vi "Initialize.vi"(8 "error in (no error)":errorcluster caption="错误输入（无错误）", 10 "VISA资源名称":refnum<visa-resource-name>, 11 "34461A 输入":refnum<class "34461A.lvclass">) -> (0 "error out":errorcluster caption="错误输出", 3 "34461A 输出":refnum<class "34461A.lvclass">)   [LabVIEW 2020, in "34461A.lvlib" / "34461A.lvclass"]
uses:
  34461A.lvclass
  <instrlib>/Agilent 3446X Series/Agilent 3446X Series.lvlib
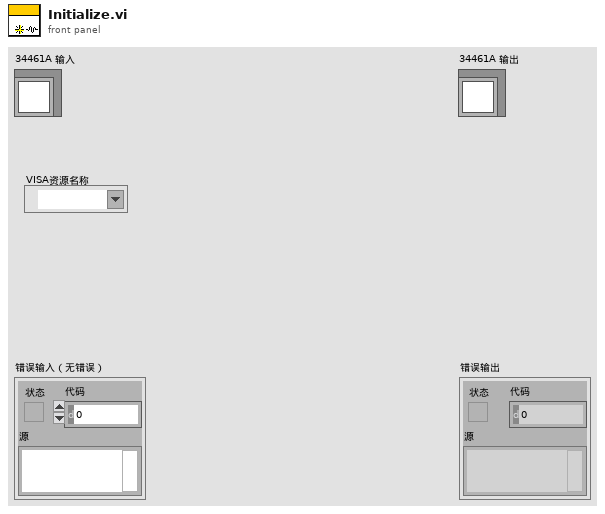
[diagram p1: front panel]
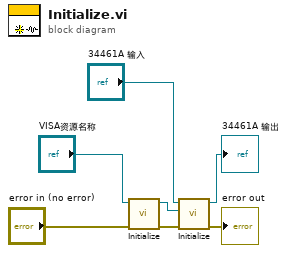
[diagram p0: block diagram]
diagram:
  n1 = call <instrlib>:"Initialize.vi"("error in (no error)"="error in (no error)", "VISA resource name"="VISA资源名称") -> ("error out"=w2:errorcluster, "VISA resource name out"=w1:refnum<visa-resource-name>)  [unwired: 8 in]
  n2 = call-parent <instrlib>:"Initialize.vi"("error in (no error)"=w2, "VISA资源名称"=w1, "数字多用表接口 输入"="34461A 输入") -> ("error out"=→"error out":errorcluster, "数字多用表接口 输出"=→"34461A 输出":refnum<class "34461A.lvclass">)  [unwired: 7 in]
